vi "publish.vi"(0 "HGF_PVObjectPublisher":refnum<class "HGF_PVObjectPublisher.lvclass">, 1 "typeDescriptor":string, 2 "data":variant, 3 "timeout in ms (-1)":i32, 5 "error in (no error)":errorcluster) -> (14 "dup HGF_PVObjectPublisher":refnum<class "HGF_PVObjectPublisher.lvclass">, 16 "rawData":variant, 17 "timed out?":bool, 19 "error out":errorcluster)   [LabVIEW 2014, in "HGF_BaseClasses.lvlib" / "HGF_PVObjectPublisher.lvclass"]
uses:
  HGF_PVObjectPublisher.lvclass
  HGF_PVPublisher/HGF_PVPublisher.lvclass
  HGF_Event/HGF_Event.lvclass
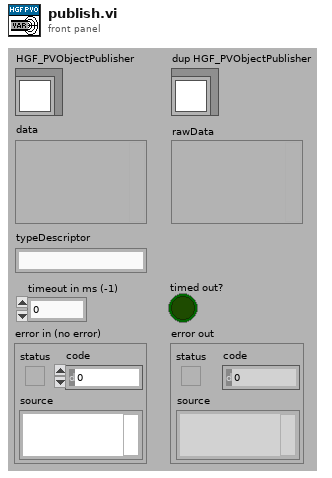
[diagram p1: front panel]
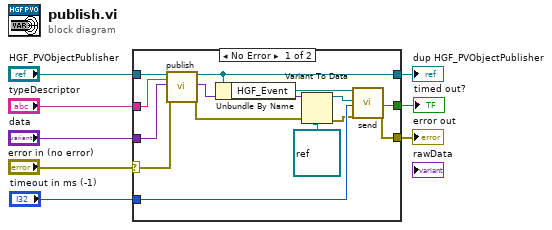
[diagram p0: block diagram]
diagram:
  n1 = case shown="No Error" "error in (no error)" {
    selector: "error in (no error)" -> [w9 w23]
    tunnel: "HGF_PVObjectPublisher" -> [w22 w24]
    tunnel: "data" -> [w21 _]
    tunnel: [w20 w24] -> w6
    tunnel: "timeout in ms (-1)" -> [w14 _]
    tunnel: [w12 w23] -> w4
    tunnel: [w11 _] -> w3
    tunnel: "typeDescriptor" -> [w10 _]
    frame No Error {
      n2 = call-parent "publish.vi"("HGF_PVPublisher"=w22, "typeDescriptor"=w10, "data"=w21, "error in (no error)"=w9) -> ("dup HGF_PVPublisher"=w20:refnum<class "HGF_PVObjectPublisher.lvclass">, "rawData"=w18:variant, "error out"=w17:errorcluster)  [unwired: 1 in, 12 out]
      n3 = Unbundle By Name(w20) -> ("HGF_Event"=w19:refnum<class "HGF_Event.lvclass">)
      n4 = Variant To Data(error in=w17, type=refnum<class> refnum, Variant=w18) -> (data=w16:refnum<class>, error out=w13:errorcluster)
      n5 = call-dynamic "send.vi"("HGF_Event"=w19, "Object"=w16, "timeout in ms (-1)"=w14, "error in (no error)"=w13) -> ("timed out?"=w11:bool, "error out"=w12:errorcluster)  [unwired: 1 in, 13 out]
    }
    frame Error {
    }
  }
  "error out" <- w4
  "dup HGF_PVObjectPublisher" <- w6
  "timed out?" <- w3
